vi "clean.vi"(8 "error in (no error)":errorcluster) -> (0 "error out":errorcluster)   [LabVIEW 2019, in "CNT90_GPIB.lvlib"]
uses:
  CNT90_GPIB.lvlib
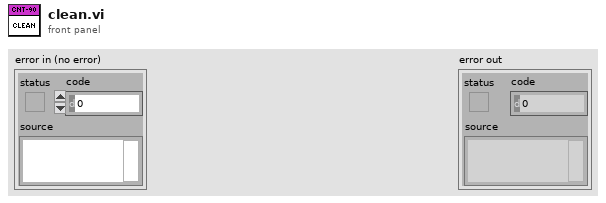
[diagram p1: front panel]
types:
  T1 = cluster{"error":bool, "code":i32, "source":string}
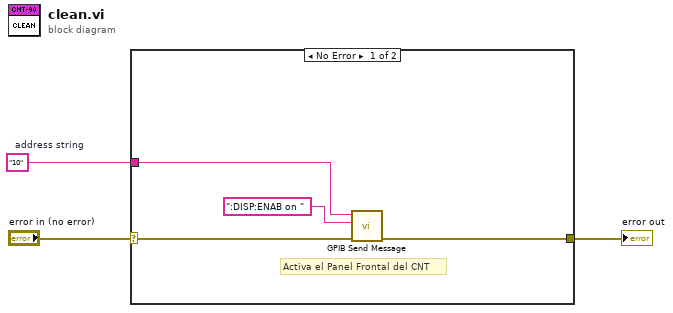
[diagram p0: block diagram]
diagram:
  w1 = "10"  # address string
  n1 = case shown="No Error" "error in (no error)" {
    selector: "error in (no error)" -> [w6 w8]
    tunnel: [w5 w8] -> w2
    tunnel: w1 -> [w4 _]
    frame No Error {
      # "Activa el Panel Frontal del CNT"
      n2 = call <instrlib>:"GPIB Send Message.vi"("address string"=w4, "write buffer"=":DISP:ENAB on ", "error in"=w6) -> ("error out"=w5:T1)  [unwired: 4 in, 2 out]
    }
    frame Error {
    }
  }
  "error out" <- w2
